vi "Global Variables.vi"() -> ()   [LabVIEW 2014]
panel:
  out "Front Lifter Fudge Factor":dbl
  out "Front Lifter Level":dbl
  in  "Calibrate?":bool
  in  "Calibrate Gyro":bool
  in  "Reset Gyro":bool
  out "Gyro Angle":dbl
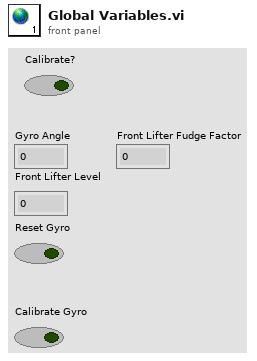
[diagram p1: front panel]
diagram:
